vi "String_Is_Number.vi"(0 "String":string) -> (1 "Number":dbl, 2 "Is Number?":bool)   [LabVIEW 2018]
doc: "Elegant method for determining if a string is a number \n\nhttps://rosettacode.org/wiki/Determine_if_a_string_is_numeric#LabVIEW\n\n10 - 8 - 2018\n\nNeed to make sure that you trim all white-space\n\nR. Sheehan 25 - 10 - 2018"
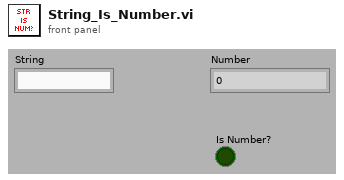
[diagram p1: front panel]
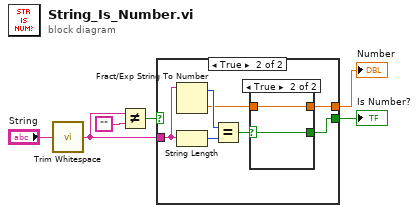
[diagram p0: block diagram]
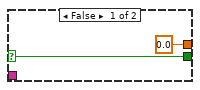
[diagram p2: hidden frame]
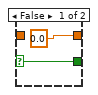
[diagram p3: hidden frame]
diagram:
  n1 = call <vilib>:"Trim Whitespace.vi"("string"="String") -> ("trimmed string"=w1:string)  [unwired: 1 in]
  n2 = Not Equal?(x=w1, y="") -> (x != y?=w3:bool)
  n3 = case shown="True" w3 {
    selector: w3 -> [w7 _]
    tunnel: w1 -> [_ w9]
    tunnel: [0.0 w11] -> w6
    tunnel: [w7 w10] -> w5
    frame False {
    }
    frame True {
      n4 = Fract/Exp String To Number(string=w9) -> (offset past number=w14:i32, number=w12:dbl)  [unwired: 3 in]
      n5 = String Length(string=w9) -> (length=w15:i32)
      n6 = Equal?(x=w14, y=w15) -> (x = y?=w13:bool)
      n7 = case shown="True" w13 {
        selector: w13 -> [w17 w18]
        tunnel: w12 -> [_ w19]
        tunnel: [0.0 w19] -> w11
        tunnel: [w17 w18] -> w10
        frame False {
        }
        frame True {
        }
      }
    }
  }
  "Number" <- w6
  "Is Number?" <- w5
